vi "WriteHeaders.vi"(0 "refnum in":refnum<file>, 5 "Match Number":u32, 7 "Date and Time":string, 9 "Battery Number":string, 11 "error in":errorcluster) -> (4 "refnum out":refnum<file>, 15 "error out":errorcluster)   [LabVIEW 2017]
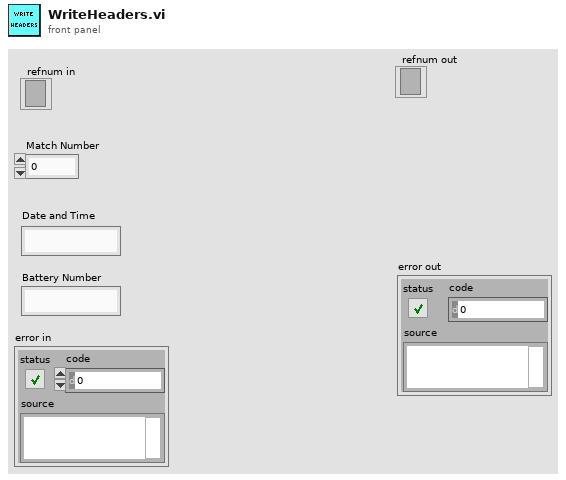
[diagram p1: front panel]
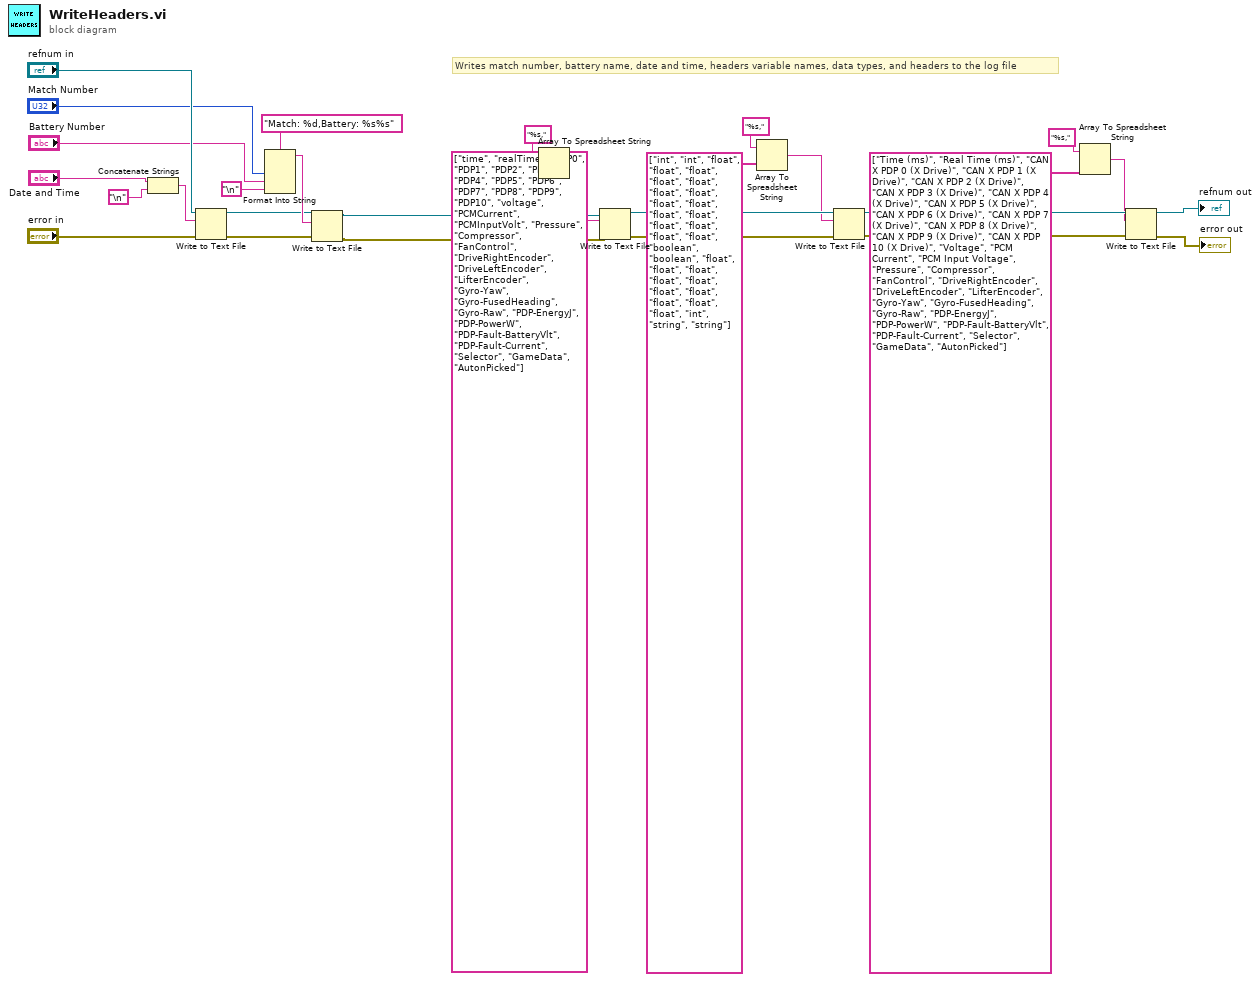
[diagram p0: block diagram]
diagram:
  # "Writes match number, battery name, date and time, headers variable names, data types, and headers to the log file"
  n1 = Concatenate Strings("Date and Time", "\n") -> (w27:string)
  n2 = Write to Text File(file (use dialog)="refnum in", text=w27, error in="error in") -> (refnum out=w21:refnum<file>, error out=w20:errorcluster)  [unwired: 1 in, 1 out]
  n3 = Format Into String(format string="Match: %d,Battery: %s%s", "Match Number", "Battery Number", "\n") -> (resulting string=w22:string)  [unwired: 2 in, 1 out]
  n4 = Write to Text File(file (use dialog)=w21, text=w22, error in=w20) -> (refnum out=w13:refnum<file>, error out=w12:errorcluster)  [unwired: 1 in, 1 out]
  n5 = Array To Spreadsheet String(array=string[] ["time", "realTime", "PDP0", "PDP1", "PDP2", "PDP3", "PDP4", "PDP5", "PDP6", "PDP7", "PDP8", "PDP9", "PDP10", "voltage", "PCMCurrent", "PCMInputVolt", "Pressure", "Compressor", "FanControl", "DriveRightEncoder", "DriveLeftEncoder", "LifterEncoder", "Gyro-Yaw", "Gyro-FusedHeading", "Gyro-Raw", "PDP-EnergyJ", "PDP-PowerW", "PDP-Fault-BatteryVlt", "PDP-Fault-Current", "Selector", "GameData", "AutonPicked"], 3:"%s," ("format string")) -> (spreadsheet string=w5:string)  [unwired: 1 in]
  n6 = Write to Text File(file (use dialog)=w13, text=w5, error in=w12) -> (refnum out=w15:refnum<file>, error out=w14:errorcluster)  [unwired: 1 in, 1 out]
  n7 = Array To Spreadsheet String(array=string[] ["int", "int", "float", "float", "float", "float", "float", "float", "float", "float", "float", "float", "float", "float", "float", "float", "float", "boolean", "boolean", "float", "float", "float", "float", "float", "float", "float", "float", "float", "float", "int", "string", "string"], 3:"%s," ("format string")) -> (spreadsheet string=w4:string)  [unwired: 1 in]
  n8 = Write to Text File(file (use dialog)=w15, text=w4, error in=w14) -> (refnum out=w9:refnum<file>, error out=w8:errorcluster)  [unwired: 1 in, 1 out]
  n9 = Array To Spreadsheet String(array=string[] ["Time (ms)", "Real Time (ms)", "CAN X PDP 0 (X Drive)", "CAN X PDP 1 (X Drive)", "CAN X PDP 2 (X Drive)", "CAN X PDP 3 (X Drive)", "CAN X PDP 4 (X Drive)", "CAN X PDP 5 (X Drive)", "CAN X PDP 6 (X Drive)", "CAN X PDP 7 (X Drive)", "CAN X PDP 8 (X Drive)", "CAN X PDP 9 (X Drive)", "CAN X PDP 10 (X Drive)", "Voltage", "PCM Current", "PCM Input Voltage", "Pressure", "Compressor", "FanControl", "DriveRightEncoder", "DriveLeftEncoder", "LifterEncoder", "Gyro-Yaw", "Gyro-FusedHeading", "Gyro-Raw", "PDP-EnergyJ", "PDP-PowerW", "PDP-Fault-BatteryVlt", "PDP-Fault-Current", "Selector", "GameData", "AutonPicked"], 3:"%s," ("format string")) -> (spreadsheet string=w3:string)  [unwired: 1 in]
  n10 = Write to Text File(file (use dialog)=w9, text=w3, error in=w8) -> (refnum out=→"refnum out":refnum<file>, error out=→"error out":errorcluster)  [unwired: 1 in, 1 out]
